vi "finishUp.vi"(8 "error in (no error)":errorcluster, 11 "WinX32Settings in":refnum<class "WinX32Settings.lvclass">) -> (0 "error out":errorcluster, 3 "WinX32Settings out":refnum<class "WinX32Settings.lvclass">)   [LabVIEW 2011, in "Tools.lvlib" / "Settings.lvlib" / "WinX32Settings.lvclass"]
uses:
  WinX32Settings.lvclass
  WinX32Settings.lvclass/WinX32Settings.ctl
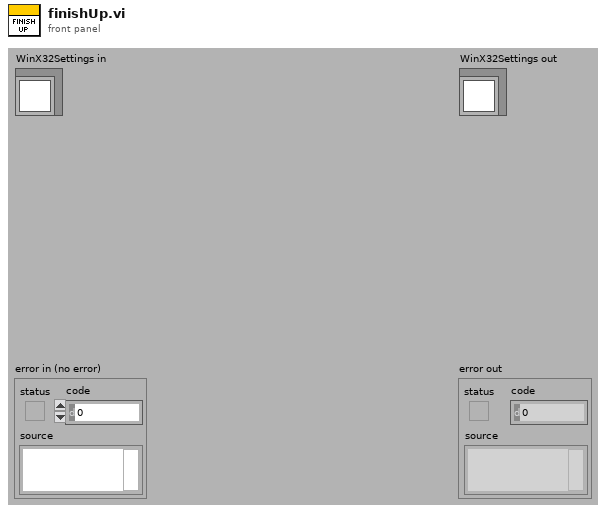
[diagram p1: front panel]
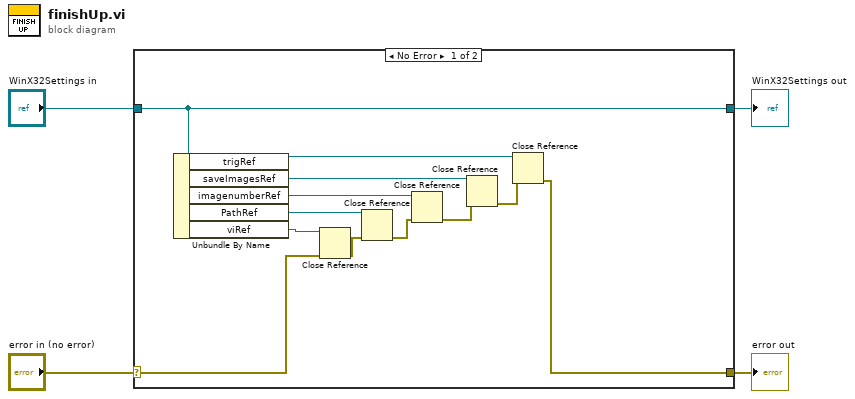
[diagram p0: block diagram]
diagram:
  n1 = case shown="No Error" "error in (no error)" {
    selector: "error in (no error)" -> [w6 w18]
    tunnel: [w5 w18] -> w3
    tunnel: [w16 w17] -> w1
    tunnel: "WinX32Settings in" -> [w16 w17]
    frame No Error {
      n2 = Unbundle By Name(w16) -> ("trigRef"=w15:refnum<vi>, "saveImagesRef"=w11:refnum<vi>, "imagenumberRef"=w12:refnum<vi>, "PathRef"=w13:refnum<vi>, "viRef"=w14:refnum<vi>)
      n3 = Close Reference(reference=w14, error in (no error)=w6) -> (error out=w7:errorcluster)
      n4 = Close Reference(reference=w13, error in (no error)=w7) -> (error out=w8:errorcluster)
      n5 = Close Reference(reference=w12, error in (no error)=w8) -> (error out=w9:errorcluster)
      n6 = Close Reference(reference=w11, error in (no error)=w9) -> (error out=w10:errorcluster)
      n7 = Close Reference(reference=w15, error in (no error)=w10) -> (error out=w5:errorcluster)
    }
    frame Error {
    }
  }
  "error out" <- w3
  "WinX32Settings out" <- w1
